vi "side_features - saveTxt.vi"() -> ()   [LabVIEW 2015]
uses:
  <vilib>/addons/_office/_exclsub.llb/font.ctl
  <vilib>/Analysis/baseanly.llb/Mean (DBL).vi
  <vilib>/Utility/file.llb/Read Delimited Spreadsheet (string).vi
  <vilib>/Utility/file.llb/Read From Spreadsheet File (string).vi
  <vilib>/addons/_office/NI_ReportGenerationToolkit.lvlib
  <vilib>/Utility/NIReport.llb/Excel/NI_Excel.lvclass
  <vilib>/vision/NI_Vision_Development_Module.lvlib
  TotalContoursConvexHull.dll
  <vilib>/Analysis/NI_AALBase.lvlib
  2-top_features_oilseed/HistProperty.dll
  PlantType.dll
panel:
  out "im_width":i32
  out "im_height":i32
  in  "The Path to save excel":path=path "E:/oilseed data/side_features"
  in  "Date Path":path=path "H:/oilseed data/date.txt"
  out "Current Path":path
  out "Current Number":string
  out "Rotated Image":T1(plugin-control)
  out "HistStat_whole":dbl[](array[numeric])
  out "PAR (perimeter-to-area ratio)":dbl
  out "SFD":sgl
  out "BW (minimum circumscribed box width)":dbl
  out "BH (minimum circumscribed box height)":dbl
  out "TPA (Total projective area)":dbl
  out "R (Rectangularity)":dbl
  out "IFD":sgl
  out "Hull area":dbl
  out "AC (Area Convexity)":dbl
  out "HWR":dbl
  in  "ROI_flower":T2={"Top"=0, "im_height"=1450, "L_left"=0, "im_width"=1680}
  out "NB (Number of blanchs)":i32
  out "FPAR (Flower perimeter-to-area ratio)":dbl
  out "FSFD":sgl
  out "FBW (Flower minimum circumscribed box width)":dbl
  out "FBH (Flower minimum circumscribed box height)":dbl
  out "YPA (Yellow projective area)":dbl
  out "FR (Flower rectangularity)":dbl
  out "FIFD":sgl
  out "FAC (Flower area Convexity)":dbl
  out "HistStat_flower":dbl[](array[numeric])
  in  "ROI_whole":T2={"Top"=90, "im_height"=1970, "L_left"=300, "im_width"=1450}
  out "FHWR":dbl
  out "GPA (Green projective area)":dbl
  out "GPAR (Green / Total)":dbl
  out "YPAR (Yellow / Total)":dbl
  out "Flower Hull Image":T1(plugin-control)
  out "Flower Hull Area":dbl
  out "Cropped Image":T1(plugin-control)
  out "Binary Image":T1(plugin-control)
  out "rgb Hull Image":T1(plugin-control)
  out "Flower Image (RGB)":T1(plugin-control)
  out "Flower Image (Label)":T1(plugin-control)
  out "PD1-6":sgl[](array[numeric])
  out "f array":dbl[](array[numeric])
  out "Combined Image":T1(plugin-control)
  in  "error in (no error) 2":errorcluster
  out "error out 2":errorcluster
  out "Image Path":path
  in  "Image Main Path":path=path "H:/oilseed data"
  out "error out":errorcluster
  in  "error in (no error)":errorcluster
  # "Digital evaluation software for oilseed rape phenotype-related traits (side-view) v1.0"
  # "测量数据"
  # "Whole plant"
  # "均值"
  # "标准差"
  # "平滑度"
  # "三阶矩"
  # "一致性"
  # "熵"
  # "Flower"
  # "Ratio"
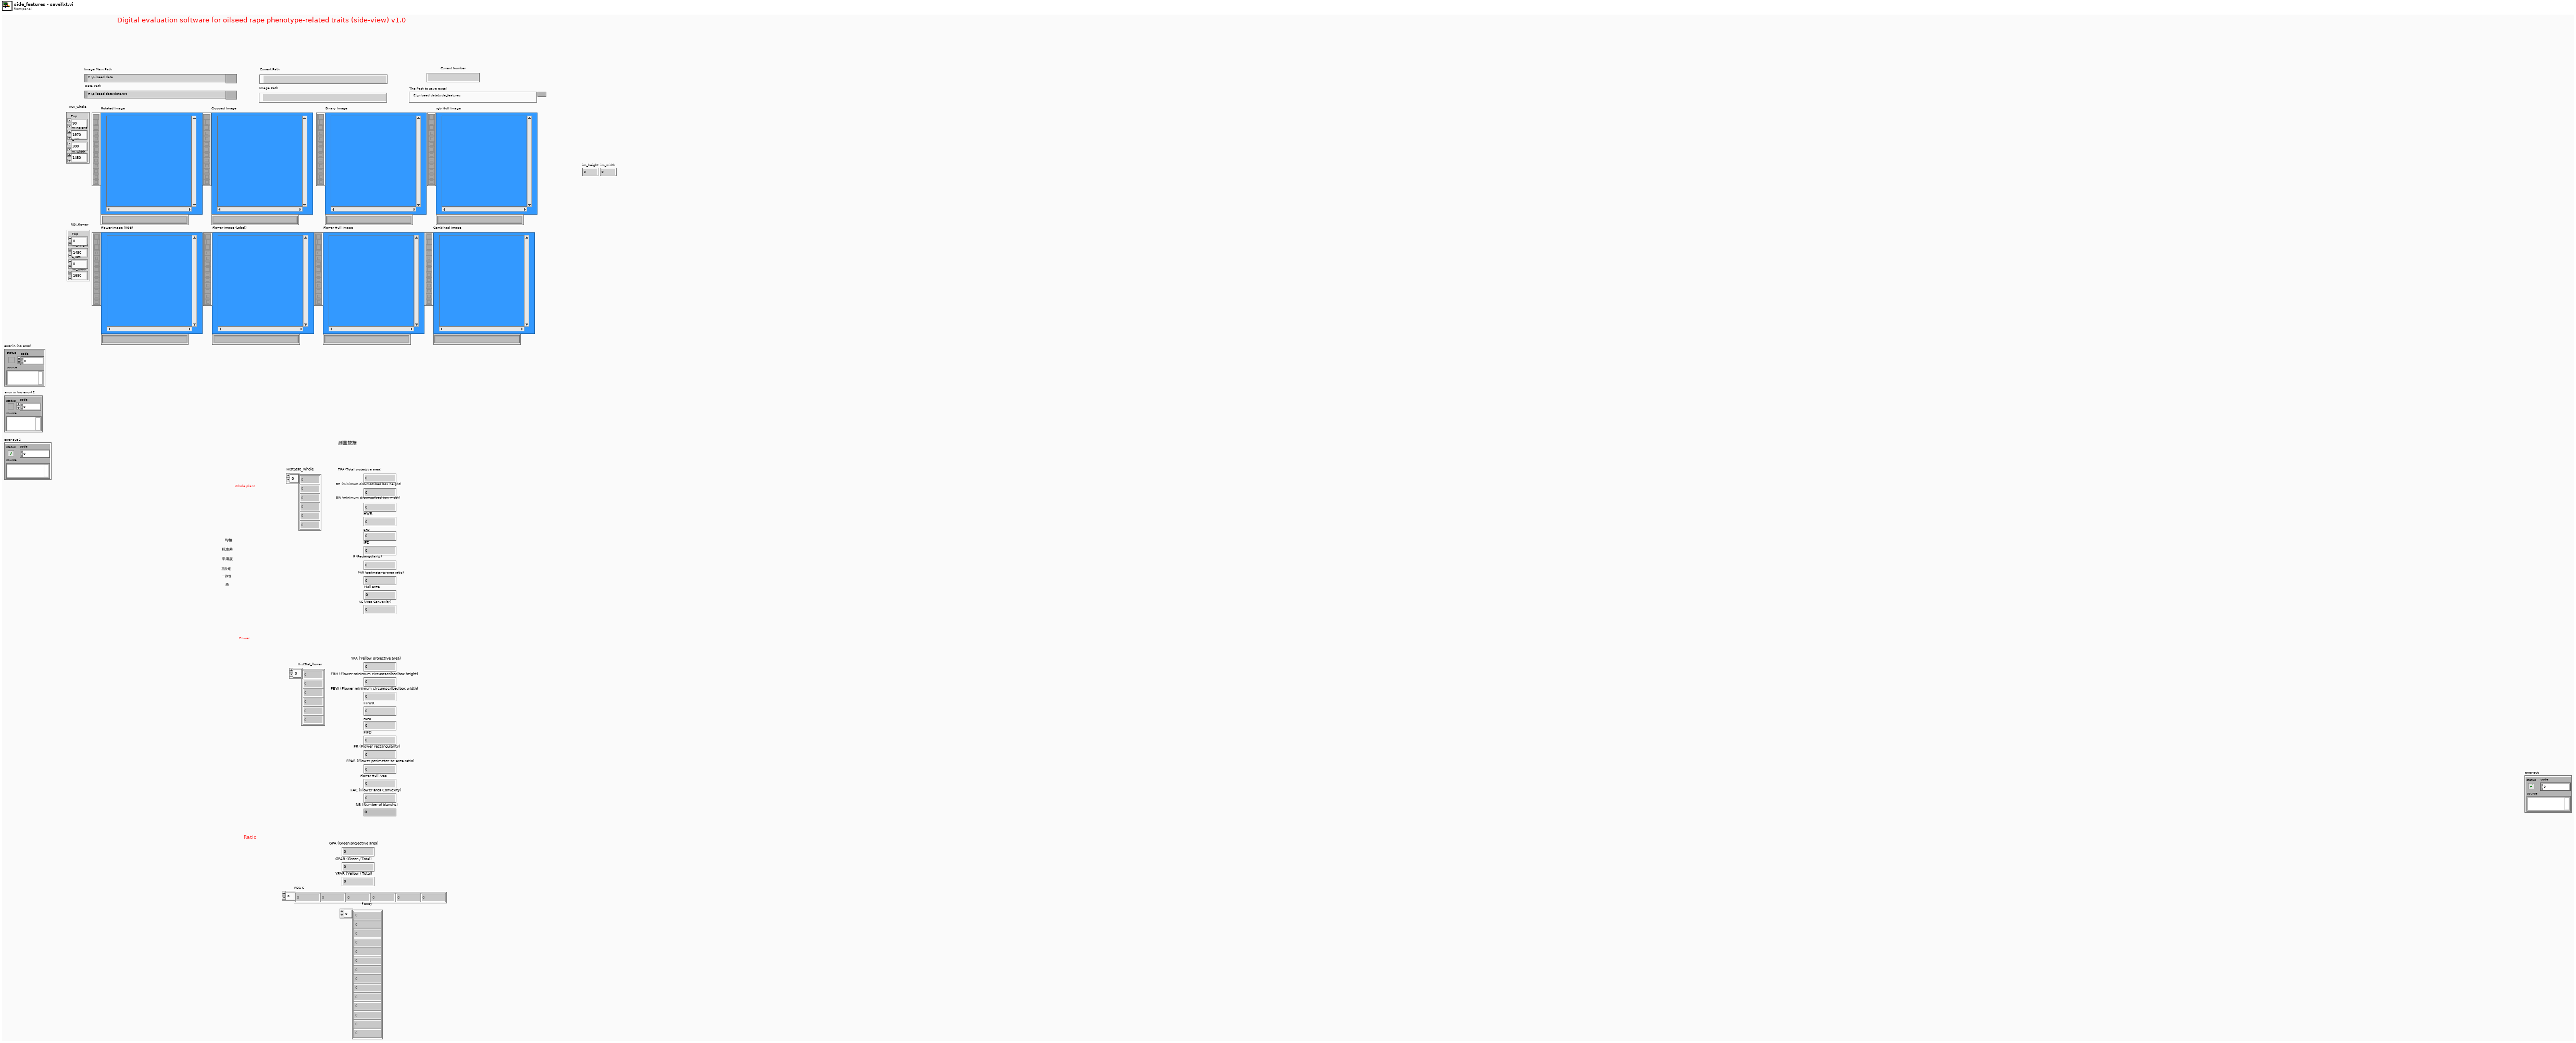
[diagram p1: front panel]
types:
  T1 = typedef "IMAQ Image.ctl" = refnum<image>
  T2 = cluster{"Top":i32, "im_height":i32, "L_left":i32, "im_width":i32}
  T3 = cluster{"report out":refnum<class "NI_report.lvclass">, "dup path":path}
  T4 = typedef "NI_ReportGenerationToolkit.lvlib/font.ctl" = cluster{"font name":string, "font size":dbl, "bold":u16, "italic":u16, "underline":u16, "strike through":u16, "font color":u32}
  T5 = typedef "Image Type" = u32
  T6 = typedef "Particle Parameters" = i32
  T7 = cluster{"String":string, "mean":dbl, "mean":dbl, "mean":dbl, "mean":dbl, "mean":dbl, "mean":dbl, "mean":dbl, "mean":dbl, "mean":dbl, "mean":dbl, "mean":dbl, "mean":dbl, "mean":dbl, "mean":dbl, "mean":dbl, "mean":dbl, "mean":dbl, "mean":dbl, "mean":dbl, "mean":dbl, "mean":dbl, "mean":dbl, "mean":dbl, "mean":dbl, "mean":dbl, "mean":dbl, "mean":dbl, "mean":dbl, "mean":dbl, "mean":dbl, "mean":dbl, "mean":dbl, "mean":dbl, "mean":dbl, "mean":dbl, "mean":dbl, "ratio":sgl[], "f array":dbl[]}
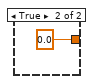
[diagram p2: hidden frame]
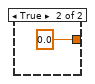
[diagram p3: hidden frame]
diagram:
  n1 = flat-sequence {
    tunnel: [w4] -> w1
    tunnel: w1 -> [w7]
    frame #0 {
      n2 = call "SheetInput (SubVI).vi"("error in (no error)"="error in (no error)", "The Path to save excel"="The Path to save excel") -> ("error out"=→"error out":errorcluster, "Cluster"=w4:T3)  [unwired: 8 in]
    }
    frame #1 {
      n3 = call-poly <vilib>:"Read Delimited Spreadsheet.vi"("file path (dialog if empty)"="Date Path") -> ("all rows"=w6:string[][])  [unwired: 9 in, 5 out]
      n4 = for {
        tunnel: "Image Main Path" -> [w19]
        tunnel: w6 -> [w17] mode=indexing
        tunnel: w7 -> [w11]
        n5 = Index Array(array=w17, index=0) -> (element=w12:string)
        n6 = Build Path(base path=w19, name or relative path=w12) -> (appended path=w13:path)
        "Image Path" <- w13
        n7 = Build Path(base path=w13, name or relative path="numbers.txt") -> (appended path=w15:path)
        n8 = call-poly <vilib>:"Read From Spreadsheet File.vi"("file path (dialog if empty)"=w15) -> ("all rows"=w14:string[][])  [unwired: 3 in, 7 out]
        n9 = for {
          tunnel: w13 -> [w542]
          tunnel: w14 -> [w543] mode=indexing
          tunnel: w11 -> [w450]
          shift-right: [w273] -> _
          shift-left: 2 -> [w84]
          w443 = 0
          w155 = T4 {"font name"="", "font size"=13.0, "bold"=0, "italic"=0, "underline"=0, "strike through"=0, "font color"=16777216} ("font")
          w534 = T5 0 items=["Grayscale (U8)", "Grayscale (I16)", "Grayscale (SGL)", "Complex (CSG)", "RGB (U32)", "HSL (U32)", "RGB (U64)", "Grayscale (U16)"] ("Image Type")
          n10 = Index Array(array=w543, index=0) -> (element=w541:string)
          n11 = local read "im_width"() -> (w24:i32)
          n12 = local read "im_height"() -> (w27:i32)
          n13 = local read "im_height"() -> (w26:i32)
          n14 = local read "im_width"() -> (w25:i32)
          n15 = call "IMAQ Create"("Image Name"="original", "Image Type"=w534) -> ("New Image"=w535:T1)  [unwired: 2 in, 2 out]
          n16 = call "IMAQ SetImageSize"("Y Resolution"=w26, "X Resolution"=w24, "Image"=w535) -> ("Image Out"=w533:T1)  [unwired: 1 in, 2 out]
          n17 = Initialize Array(sgl 0.0 ("element"), w27, w25) -> (w538:sgl[][])
          n18 = Increment(x=w84) -> (x+1=w273:i32)
          n19 = for {
            N: 15 -> [_]
            tunnel: w542 -> [w633]
            tunnel: w541 -> [w546]
            shift-right: [w599] -> w537
            shift-left: w538 -> [w602]
            shift-right: [w597] -> w458
            shift-left: w533 -> [w598]
            tunnel: [w595] -> w532 mode=indexing
            tunnel: [w594] -> w531 mode=indexing
            tunnel: [w593] -> w530 mode=indexing
            tunnel: [w592] -> w529 mode=indexing
            tunnel: [w591] -> w528 mode=indexing
            tunnel: [w590] -> w527 mode=indexing
            tunnel: [w589] -> w520 mode=indexing
            tunnel: [w588] -> w518 mode=indexing
            tunnel: [w587] -> w517 mode=indexing
            tunnel: [w586] -> w514 mode=indexing
            tunnel: [w585] -> w512 mode=indexing
            tunnel: [w584] -> w511 mode=indexing
            tunnel: [w583] -> w510 mode=indexing
            tunnel: [w582] -> w509 mode=indexing
            tunnel: [w581] -> w508 mode=indexing
            tunnel: [w580] -> w507 mode=indexing
            tunnel: [w578] -> w500 mode=indexing
            tunnel: [w577] -> w499 mode=indexing
            tunnel: [w576] -> w498 mode=indexing
            tunnel: [w575] -> w497 mode=indexing
            tunnel: [w574] -> w496 mode=indexing
            tunnel: [w573] -> w495 mode=indexing
            tunnel: [w554] -> w488 mode=indexing
            tunnel: [w572] -> w487 mode=indexing
            tunnel: [w571] -> w486 mode=indexing
            tunnel: [w570] -> w485 mode=indexing
            tunnel: [w569] -> w484 mode=indexing
            tunnel: [w568] -> w483 mode=indexing
            tunnel: [w567] -> w482 mode=indexing
            tunnel: [w566] -> w481 mode=indexing
            tunnel: [w553] -> w480 mode=indexing
            tunnel: [w552] -> w479 mode=indexing
            tunnel: [w565] -> w478 mode=indexing
            tunnel: [w564] -> w466 mode=indexing
            tunnel: [w563] -> w465 mode=indexing
            tunnel: [w562] -> w464 mode=indexing
            tunnel: [w546] -> w456 mode=indexing
            i -> [w545]
            w561 = T6[] [35] items=["Center of Mass X", "Center of Mass Y", "First Pixel X", "First Pixel Y", "Bounding Rect Left", "Bounding Rect Top", "Bounding Rect Right", "Bounding Rect Bottom", "Max Feret Diameter Start X", "Max Feret Diameter Start Y", "Max Feret Diameter End X", "Max Feret Diameter End Y", "Max Horiz. Segment Length Left", "Max Horiz. Segment Length Right", "Max Horiz. Segment Length Row", "-", "Bounding Rect Width", "Bounding Rect Height", "Bounding Rect Diagonal", "Perimeter", "Convex Hull Perimeter", "Holes' Perimeter", "Max Feret Diameter", "Equivalent Ellipse Major Axis", "Equivalent Ellipse Minor Axis", "Equivalent Ellipse Minor Axis (Feret)", "Equivalent Rect Long Side", "Equivalent Rect Short Side", "Equivalent Rect Diagonal", "Equivalent Rect Short Side (Feret)", "Average Horiz. Segment Length", "Average Vert. Segment Length", "Hydraulic Radius", "Waddel Disk Diameter", "-", "Area", "Holes' Area", "Particle & Holes' Area", "Convex Hull Area", "Image Area", "-", "Number of Holes", "Number of Horiz. Segments", "Number of Vert. Segments", "-", "Orientation", "Max Feret Diameter Orientation", "-", "% Area/Image Area", "% Area/(Particle & Holes' Area)", "Ratio of Equivalent Ellipse Axes", "Ratio of Equivalent Rect Sides", "-", "Elongation Factor", "Compactness Factor", "Heywood Circularity Factor", "Type Factor", "-", "Sum X", "Sum Y", "Sum XX", "Sum XY", "Sum YY", "Sum XXX", "Sum XXY", "Sum XYY", "Sum YYY", "-", "Moment of Inertia XX", "Moment of Inertia XY", "Moment of Inertia YY", "Moment of Inertia XXX", "Moment of Inertia XXY", "Moment of Inertia XYY", "Moment of Inertia YYY", "Norm. Moment of Inertia XX", "Norm. Moment of Inertia XY", "Norm. Moment of Inertia YY", "Norm. Moment of Inertia XXX", "Norm. Moment of Inertia XXY", "Norm. Moment of Inertia XYY", "Norm. Moment of Inertia YYY", "Hu Moment 1", "Hu Moment 2", "Hu Moment 3", "Hu Moment 4", "Hu Moment 5", "Hu Moment 6", "Hu Moment 7"] ("Pixel Measurements")
            w618 = u32 4 items=["Grayscale (U8)", "Grayscale (I16)", "Grayscale (SGL)", "Complex (CSG)", "RGB (U32)", "HSL (U32)", "RGB (U64)"] ("Image Type")
            w631 = T5 4 items=["Grayscale (U8)", "Grayscale (I16)", "Grayscale (SGL)", "Complex (CSG)", "RGB (U32)", "HSL (U32)", "RGB (U64)", "Grayscale (U16)"] ("Image Type")
            w638 = T5 4 items=["Grayscale (U8)", "Grayscale (I16)", "Grayscale (SGL)", "Complex (CSG)", "RGB (U32)", "HSL (U32)", "RGB (U64)", "Grayscale (U16)"] ("Image Type")
            n20 = Number To Decimal String(number=w545) -> (decimal integer string=w635:string)  [unwired: 1 out]
            n21 = Less Or Equal?(x=w545, y=u32 7) -> (x <= y?=w600:bool)
            n22 = Concatenate Strings(w546, "_" ("string"), w635, ".png" ("string")) -> (w627:string)
            "Current Number" <- w627
            n23 = call "IMAQ Create"("Image Name"="rgb", "Image Type"=w638) -> ("New Image"=w639:T1)  [unwired: 2 in, 2 out]
            n24 = Build Path(base path=w633, name or relative path=w627) -> (appended path=w634:path)
            "Current Path" <- w634
            n25 = call "IMAQ Create"("Image Name"="1", "Image Type"=w631) -> ("New Image"=w629:T1)  [unwired: 2 in, 2 out]
            n26 = call "IMAQ ReadFile"("File Path"=w634, "Image"=w639) -> ("Image Out"=w626:T1)  [unwired: 3 in, 6 out]
            n27 = call "IMAQ Rotate"("Maintain Size"=FALSE, "Angle (degrees)"=sgl 90.0, "Image Dst"=w629, "Image Src"=w626) -> ("Image Dst Out"=w616:T1)  [unwired: 4 in, 3 out]
            "Rotated Image" <- w616
            n28 = Unbundle By Name("ROI_whole") -> ("Top"=w622:i32, "im_height"=w623:i32, "L_left"=w624:i32, "im_width"=w625:i32)
            "im_height" <- w623
            "im_width" <- w625
            n29 = call "IMAQ ColorImageToArray"("Image"=w616) -> ("Image Pixels (U32)"=w621:u32[][])  [unwired: 2 in, 3 out]
            n30 = Array Subset(array=w621, index (row)=w622, length (row)=w623, index (col)=w624, length (col)=w625) -> (w620:u32[][])
            n31 = call "IMAQ Create"("Image Name"="ROI123", "Image Type"=w618) -> ("New Image"=w617:T1)  [unwired: 2 in, 2 out]
            n32 = call "IMAQ ArrayToColorImage"("Image Pixels (U32)"=w620, "Image"=w617) -> ("Image Out"=w551:T1)  [unwired: 2 in, 2 out]
            "Cropped Image" <- w551
            n33 = call "Flower segement(SubVI).vi"("Image in"=w551, "ROI 上半部分 2"="ROI_flower") -> ("黄色分量（油菜花）二值图"=w614:T1, "黄色分量（油菜花）"=→"Flower Image (RGB)":T1, "黄色分量（油菜花）Gray"=w604:T1, "Number of Particles"=w565:i32, "RGB花标记"=w547:T1)
            "NB (Number of blanchs)" <- w565
            "Flower Image (Label)" <- w547
            n34 = call "Segement(SubVI).vi"("Image in"=w551) -> ("Binary Image"=w550:T1)
            "Binary Image" <- w550
            n35 = call "IMAQ Particle Analysis"("Pixel Measurements"=w561, "Image"=w547) -> ("Particle Measurements (Pixels)"=w560:dbl[][])  [unwired: 3 in, 6 out]
            n36 = call "HistStat(SubVI).vi"("Binary Image"=w550, "Original Image"=w551) -> ("HistStat"=w596:dbl[])  [unwired: 1 out]
            "HistStat_whole" <- w596
            n37 = call "IMAQ ImageToArray"("Image"=w604) -> ("Image Pixels (U8)"=w605:u8[][])  [unwired: 2 in, 5 out]
            n38 = call "IMAQ GetImageSize"("Image"=w604) -> ("Y Resolution"=w608:i32, "X Resolution"=w609:i32)  [unwired: 1 in, 3 out]
            n39 = case shown="True" w600 {
              tunnel: w550 -> [_ w664]
              tunnel: w602 -> [w660 w663]
              tunnel: [w660 w662] -> w599
              frame False {
              }
              frame True {
                n40 = call "IMAQ ImageToArray"("Image"=w664) -> ("Image Pixels (U8)"=w667:u8[][])  [unwired: 2 in, 5 out]
                n41 = call "IMAQ GetImageSize"("Image"=w664) -> ("Y Resolution"=w665:i32, "X Resolution"=w666:i32)  [unwired: 1 in, 3 out]
                n42 = dll-call lib="H:/3-side_features_oilseed/PlantType.dll" fn="CalLeafDens"("bw"=w667, "row"=w665, "col"=w666, "GridSize"=5, "dens"=w663) -> ("dens"=w662:sgl[][])  [unwired: 7 in, 3 out]
              }
            }
            n43 = call "IMAQ Add"("Image Src A"=w598, "Image Src B"=w550) -> ("Image Dst Out"=w597:T1)  [unwired: 3 in, 3 out]
            n44 = Add Array Elements(numeric array=w560) -> (sum=w559:dbl)
            n45 = disable-structure shown="Enabled" {
              disable-tunnel: w605 -> [w672 w673]
              disable-tunnel: u8 8 ("y") -> [w671 _]
              disable-tunnel: [w668 w673] -> w607
              frame Enabled {
                n46 = Divide(x=w672, y=w671) -> (x/y=w670:dbl[][])
                n47 = Round Toward -Infinity(1:w670) -> (0:w669:dbl[][])
                n48 = To Unsigned Byte Integer(number=w669) -> (unsigned 8bit integer=w668:u8[][])
              }
              frame Disabled {
              }
            }
            n49 = Less Or Equal?(x=w559, y=50.0) -> (x <= y?=w557:bool)
            n50 = case shown="False" w557 {
              tunnel: w547 -> [w647 _]
              tunnel: [w646 0.0 ("areaSum")] -> w553
              frame False {
                w653 = T5 4 items=["Grayscale (U8)", "Grayscale (I16)", "Grayscale (SGL)", "Complex (CSG)", "RGB (U32)", "HSL (U32)", "RGB (U64)", "Grayscale (U16)"] ("Image Type")
                n51 = call "IMAQ ImageToArray"("Image"=w647) -> ("Image Pixels (U8)"=w658:u8[][])  [unwired: 2 in, 5 out]
                n52 = call "IMAQ GetImageSize"("Image"=w647) -> ("Y Resolution"=w656:i32, "X Resolution"=w657:i32)  [unwired: 1 in, 3 out]
                n53 = Initialize Array(u8 0 ("element"), w656, w657) -> (w648:u8[][])
                n54 = Initialize Array(u32 0 ("element"), w656, w657) -> (w651:u32[][])
                n55 = dll-call lib="H:/3-side_features_oilseed/TotalContoursConvexHull.dll" fn="TotalContoursConvexHull"("src"=w658, "width"=w657, "height"=w656, "bwhullimage"=w648, "rgbhullimage"=w651) -> ("areaSum"=w646:dbl, "rgbhullimage"=w654:u32[][])  [unwired: 7 in, 2 out]
                n56 = call "IMAQ Create"("Image Name"="rgbhullimage_flower", "Image Type"=w653) -> ("New Image"=w655:T1)  [unwired: 2 in, 2 out]
                n57 = call "IMAQ ArrayToColorImage"("Image Pixels (U32)"=w654, "Image"=w655) -> ("Image Out"=→"Flower Hull Image":T1)  [unwired: 2 in, 2 out]
              }
              frame True {
              }
            }
            "Flower Hull Area" <- w553
            n58 = Initialize Array(0.0 ("element"), 6 ("dimension size")) -> (w612:dbl[])
            n59 = dll-call lib="H:/2-top_features_oilseed/HistProperty.dll" fn="HistProperty"("Im"=w607, "row"=w608, "col"=w609, "G"=32, "HistStat"=w612) -> ("HistStat"=w579:dbl[])  [unwired: 7 in, 3 out]
            "HistStat_flower" <- w579
            n60 = call "Feature_flower(SubVI).vi"("黄色分量（油菜花）二值图"=w614) -> ("SF 3"=w567:dbl, "IFD 2"=w568:sgl, "SFD 2"=w569:sgl, "SH 2"=w572:dbl, "SW 2"=w571:dbl, "SE 2"=w566:dbl, "SA"=w554:dbl)  [unwired: 1 out]
            "FPAR (Flower perimeter-to-area ratio)" <- w566
            "FSFD" <- w569
            "FBW (Flower minimum circumscribed box width)" <- w571
            "FBH (Flower minimum circumscribed box height)" <- w572
            "YPA (Yellow projective area)" <- w554
            "FR (Flower rectangularity)" <- w567
            "FIFD" <- w568
            n61 = Equal?(x=w553, y=0.0) -> (x = y?=w556:bool)
            n62 = Divide(x=w572, y=w571) -> (x/y=w570:dbl)
            "FHWR" <- w570
            n63 = case shown="False" w556 {
              tunnel: w554 -> [w643 _]
              tunnel: w553 -> [w642 _]
              tunnel: [w641 0.0] -> w552
              frame False {
                n64 = Divide(x=w643, y=w642) -> (x/y=w641:dbl)
              }
              frame True {
              }
            }
            "FAC (Flower area Convexity)" <- w552
            n65 = call "Feature_whole(SubVI).vi"("Binary Image"=w550) -> ("SE"=w582:dbl, "rgb Hull Image 2"=→"rgb Hull Image":T1, "SA"=w589:dbl, "SFD"=w585:sgl, "Hull area"=w581:dbl, "SW"=w587:dbl, "SF 2"=w580:dbl, "IFD"=w584:sgl, "SF"=w583:dbl, "SH"=w588:dbl)  [unwired: 5 out]
            "PAR (perimeter-to-area ratio)" <- w582
            "SFD" <- w585
            "BW (minimum circumscribed box width)" <- w587
            "BH (minimum circumscribed box height)" <- w588
            "TPA (Total projective area)" <- w589
            "R (Rectangularity)" <- w583
            "IFD" <- w584
            "Hull area" <- w581
            "AC (Area Convexity)" <- w580
            n66 = Subtract(x=w589, y=w554) -> (x-y=w564:dbl)
            "GPA (Green projective area)" <- w564
            n67 = Divide(x=w554, y=w589) -> (x/y=w562:dbl)
            "YPAR (Yellow / Total)" <- w562
            n68 = Divide(x=w588, y=w587) -> (x/y=w586:dbl)
            "HWR" <- w586
            n69 = Divide(x=w564, y=w589) -> (x/y=w563:dbl)
            "GPAR (Green / Total)" <- w563
            n70 = Index Array(array=w596) -> (element #1=w595:dbl, element #2=w594:dbl, element #3=w593:dbl, element #4=w592:dbl, element #5=w591:dbl, element #6=w590:dbl)  [unwired: 6 in]
            n71 = Index Array(array=w579) -> (element #1=w578:dbl, element #2=w577:dbl, element #3=w576:dbl, element #4=w575:dbl, element #5=w574:dbl, element #6=w573:dbl)  [unwired: 6 in]
          }
          "Combined Image" <- w458
          n72 = call-poly <vilib>:"Mean.vi"("X"=w532) -> ("mean"=w526:dbl)  [unwired: 1 out]
          n73 = call-poly <vilib>:"Mean.vi"("X"=w531) -> ("mean"=w525:dbl)  [unwired: 1 out]
          n74 = call-poly <vilib>:"Mean.vi"("X"=w530) -> ("mean"=w524:dbl)  [unwired: 1 out]
          n75 = call-poly <vilib>:"Mean.vi"("X"=w529) -> ("mean"=w523:dbl)  [unwired: 1 out]
          n76 = call-poly <vilib>:"Mean.vi"("X"=w528) -> ("mean"=w522:dbl)  [unwired: 1 out]
          n77 = call-poly <vilib>:"Mean.vi"("X"=w527) -> ("mean"=w521:dbl)  [unwired: 1 out]
          n78 = call-poly <vilib>:"Mean.vi"("X"=w480) -> ("mean"=w469:dbl)  [unwired: 1 out]
          n79 = call-poly <vilib>:"Mean.vi"("X"=w479) -> ("mean"=w468:dbl)  [unwired: 1 out]
          n80 = call-poly <vilib>:"Mean.vi"("X"=w478) -> ("mean"=w467:dbl)  [unwired: 1 out]
          n81 = call-poly <vilib>:"Mean.vi"("X"=w500) -> ("mean"=w494:dbl)  [unwired: 1 out]
          n82 = call-poly <vilib>:"Mean.vi"("X"=w499) -> ("mean"=w493:dbl)  [unwired: 1 out]
          n83 = call-poly <vilib>:"Mean.vi"("X"=w498) -> ("mean"=w492:dbl)  [unwired: 1 out]
          n84 = call-poly <vilib>:"Mean.vi"("X"=w497) -> ("mean"=w491:dbl)  [unwired: 1 out]
          n85 = call-poly <vilib>:"Mean.vi"("X"=w496) -> ("mean"=w490:dbl)  [unwired: 1 out]
          n86 = call-poly <vilib>:"Mean.vi"("X"=w495) -> ("mean"=w489:dbl)  [unwired: 1 out]
          n87 = call-poly <vilib>:"Mean.vi"("X"=w486) -> ("mean"=w475:dbl)  [unwired: 1 out]
          n88 = call-poly <vilib>:"Mean.vi"("X"=w485) -> ("mean"=w474:dbl)  [unwired: 1 out]
          n89 = call-poly <vilib>:"Mean.vi"("X"=w487) -> ("mean"=w476:dbl)  [unwired: 1 out]
          n90 = call-poly <vilib>:"Mean.vi"("X"=w484) -> ("mean"=w473:dbl)  [unwired: 1 out]
          n91 = call-poly <vilib>:"Mean.vi"("X"=w482) -> ("mean"=w471:dbl)  [unwired: 1 out]
          n92 = call-poly <vilib>:"Mean.vi"("X"=w483) -> ("mean"=w472:dbl)  [unwired: 1 out]
          n93 = call-poly <vilib>:"Mean.vi"("X"=w481) -> ("mean"=w470:dbl)  [unwired: 1 out]
          n94 = call "RatioCalculation.vi"("dens"=w537) -> ("ratio"=w460:sgl[])  [unwired: 2 out]
          "PD1-6" <- w460
          n95 = call-poly <vilib>:"Mean.vi"("X"=w488) -> ("mean"=w477:dbl)  [unwired: 1 out]
          n96 = call-poly <vilib>:"Mean.vi"("X"=w466) -> ("mean"=w463:dbl)  [unwired: 1 out]
          n97 = call-poly <vilib>:"Mean.vi"("X"=w464) -> ("mean"=w461:dbl)  [unwired: 1 out]
          n98 = call-poly <vilib>:"Mean.vi"("X"=w509) -> ("mean"=w503:dbl)  [unwired: 1 out]
          n99 = call-poly <vilib>:"Mean.vi"("X"=w465) -> ("mean"=w462:dbl)  [unwired: 1 out]
          n100 = call-poly <vilib>:"Mean.vi"("X"=w520) -> ("mean"=w519:dbl)  [unwired: 1 out]
          n101 = call-poly <vilib>:"Mean.vi"("X"=w512) -> ("mean"=w506:dbl)  [unwired: 1 out]
          n102 = call-poly <vilib>:"Mean.vi"("X"=w517) -> ("mean"=w515:dbl)  [unwired: 1 out]
          n103 = call-poly <vilib>:"Mean.vi"("X"=w514) -> ("mean"=w513:dbl)  [unwired: 1 out]
          n104 = call-poly <vilib>:"Mean.vi"("X"=w518) -> ("mean"=w516:dbl)  [unwired: 1 out]
          n105 = call-poly <vilib>:"Mean.vi"("X"=w510) -> ("mean"=w504:dbl)  [unwired: 1 out]
          n106 = call-poly <vilib>:"Mean.vi"("X"=w511) -> ("mean"=w505:dbl)  [unwired: 1 out]
          n107 = call-poly <vilib>:"Mean.vi"("X"=w507) -> ("mean"=w501:dbl)  [unwired: 1 out]
          n108 = call-poly <vilib>:"Mean.vi"("X"=w508) -> ("mean"=w502:dbl)  [unwired: 1 out]
          n109 = call "FreqCalculation.vi"("Acc Image"=w458) -> ("f array"=w459:dbl[])  [unwired: 2 out]
          "f array" <- w459
          n110 = Index Array(array=w456, index=0) -> (element=w454:string)
          n111 = Bundle("String"=w454, "mean"=w526, "mean"=w525, "mean"=w524, "mean"=w523, "mean"=w522, "mean"=w521, "mean"=w519, "mean"=w516, "mean"=w515, "mean"=w513, "mean"=w506, "mean"=w505, "mean"=w504, "mean"=w503, "mean"=w502, "mean"=w501, "mean"=w494, "mean"=w493, "mean"=w492, "mean"=w491, "mean"=w490, "mean"=w489, "mean"=w477, "mean"=w476, "mean"=w475, "mean"=w474, "mean"=w473, "mean"=w472, "mean"=w471, "mean"=w470, "mean"=w469, "mean"=w468, "mean"=w467, "mean"=w463, "mean"=w462, "mean"=w461, "ratio"=w460, "f array"=w459) -> (w457:T7)  [unwired: 1 in]
          n112 = Bundle(w84, w443) -> (w452:cluster{i32, i32})  [unwired: 1 in]
          n113 = Unbundle(w450) -> ("report out"=w449:refnum<class "NI_report.lvclass">, "dup path"=w21:path)
          n114 = Unbundle(w457) -> ("String"=w453:string, "mean"=w447:dbl, "mean"=w428:dbl, "mean"=w426:dbl, "mean"=w424:dbl, "mean"=w422:dbl, "mean"=w420:dbl, "mean"=w418:dbl, "mean"=w351:dbl, "mean"=w350:dbl, "mean"=w349:dbl, "mean"=w348:dbl, "mean"=w345:dbl, "mean"=w344:dbl, "mean"=w343:dbl, "mean"=w342:dbl, "mean"=w341:dbl, "mean"=w340:dbl, "mean"=w339:dbl, "mean"=w338:dbl, "mean"=w337:dbl, "mean"=w332:dbl, "mean"=w331:dbl, "mean"=w330:dbl, "mean"=w264:dbl, "mean"=w263:dbl, "mean"=w262:dbl, "mean"=w261:dbl, "mean"=w260:dbl, "mean"=w259:dbl, "mean"=w258:dbl, "mean"=w257:dbl, "mean"=w256:dbl, "mean"=w255:dbl, "mean"=w254:dbl, "mean"=w253:dbl, "mean"=w252:dbl, "ratio"=w232:sgl[], "f array"=w216:dbl[])
          n115 = Increment(x=w443) -> (x+1=w410:i32)
          n116 = Index Array(array=w232, index=5) -> (element=w231:sgl)
          n117 = Index Array(array=w232, index=4) -> (element=w233:sgl)
          n118 = Index Array(array=w232, index=3) -> (element=w236:sgl)
          n119 = Index Array(array=w232, index=2) -> (element=w243:sgl)
          n120 = Index Array(array=w232, index=1) -> (element=w244:sgl)
          n121 = Index Array(array=w232, index=0) -> (element=w250:sgl)
          n122 = Index Array(array=w216, index=9) -> (element=w145:dbl)
          n123 = Index Array(array=w216, index=8) -> (element=w146:dbl)
          n124 = Index Array(array=w216, index=7) -> (element=w147:dbl)
          n125 = Index Array(array=w216, index=6) -> (element=w148:dbl)
          n126 = Index Array(array=w216, index=5) -> (element=w149:dbl)
          n127 = Index Array(array=w216, index=4) -> (element=w150:dbl)
          n128 = Index Array(array=w216, index=3) -> (element=w151:dbl)
          n129 = Index Array(array=w216, index=2) -> (element=w152:dbl)
          n130 = Index Array(array=w216, index=1) -> (element=w153:dbl)
          n131 = Index Array(array=w216, index=0) -> (element=w154:dbl)
          n132 = Index Array(array=w216, index=13) -> (element=w141:dbl)
          n133 = Index Array(array=w216, index=12) -> (element=w142:dbl)
          n134 = Index Array(array=w216, index=11) -> (element=w143:dbl)
          n135 = Index Array(array=w216, index=10) -> (element=w144:dbl)
          n136 = call <vilib>:"Excel Easy Text.vi"("report in"=w449, "border? (F)"=FALSE, "font"=w155, "text"=w453, "start (-1, -1)"=w452, "error in (no error)"="error in (no error) 2") -> ("report out"=w444:refnum<class "NI_report.lvclass">, "error out"=w441:errorcluster)  [unwired: 5 in, 3 out]
          n137 = Bundle(w84, w410) -> (w442:cluster{i32, i32})  [unwired: 1 in]
          n138 = Number To Fractional String(number=w447) -> (F-format string=w446:string)  [unwired: 3 in]
          n139 = Increment(x=w410) -> (x+1=w138:i32)
          n140 = call <vilib>:"Excel Easy Text.vi"("report in"=w444, "border? (F)"=FALSE, "font"=w155, "text"=w446, "start (-1, -1)"=w442, "error in (no error)"=w441) -> ("report out"=w434:refnum<class "NI_report.lvclass">, "error out"=w440:errorcluster)  [unwired: 5 in, 3 out]
          n141 = Bundle(w84, w138) -> (w409:cluster{i32, i32})  [unwired: 1 in]
          n142 = Number To Fractional String(number=w428) -> (F-format string=w427:string)  [unwired: 3 in]
          n143 = Increment(x=w138) -> (x+1=w137:i32)
          n144 = call <vilib>:"Excel Easy Text.vi"("report in"=w434, "border? (F)"=FALSE, "font"=w155, "text"=w427, "start (-1, -1)"=w409, "error in (no error)"=w440) -> ("report out"=w433:refnum<class "NI_report.lvclass">, "error out"=w439:errorcluster)  [unwired: 5 in, 3 out]
          n145 = Bundle(w84, w137) -> (w81:cluster{i32, i32})  [unwired: 1 in]
          n146 = Number To Fractional String(number=w426) -> (F-format string=w425:string)  [unwired: 3 in]
          n147 = Increment(x=w137) -> (x+1=w136:i32)
          n148 = call <vilib>:"Excel Easy Text.vi"("report in"=w433, "border? (F)"=FALSE, "font"=w155, "text"=w425, "start (-1, -1)"=w81, "error in (no error)"=w439) -> ("report out"=w432:refnum<class "NI_report.lvclass">, "error out"=w438:errorcluster)  [unwired: 5 in, 3 out]
          n149 = Bundle(w84, w136) -> (w80:cluster{i32, i32})  [unwired: 1 in]
          n150 = Number To Fractional String(number=w424) -> (F-format string=w423:string)  [unwired: 3 in]
          n151 = Increment(x=w136) -> (x+1=w135:i32)
          n152 = call <vilib>:"Excel Easy Text.vi"("report in"=w432, "border? (F)"=FALSE, "font"=w155, "text"=w423, "start (-1, -1)"=w80, "error in (no error)"=w438) -> ("report out"=w431:refnum<class "NI_report.lvclass">, "error out"=w437:errorcluster)  [unwired: 5 in, 3 out]
          n153 = Bundle(w84, w135) -> (w79:cluster{i32, i32})  [unwired: 1 in]
          n154 = Number To Fractional String(number=w422) -> (F-format string=w421:string)  [unwired: 3 in]
          n155 = Increment(x=w135) -> (x+1=w134:i32)
          n156 = call <vilib>:"Excel Easy Text.vi"("report in"=w431, "border? (F)"=FALSE, "font"=w155, "text"=w421, "start (-1, -1)"=w79, "error in (no error)"=w437) -> ("report out"=w430:refnum<class "NI_report.lvclass">, "error out"=w436:errorcluster)  [unwired: 5 in, 3 out]
          n157 = Bundle(w84, w134) -> (w78:cluster{i32, i32})  [unwired: 1 in]
          n158 = Number To Fractional String(number=w420) -> (F-format string=w419:string)  [unwired: 3 in]
          n159 = Increment(x=w134) -> (x+1=w133:i32)
          n160 = call <vilib>:"Excel Easy Text.vi"("report in"=w430, "border? (F)"=FALSE, "font"=w155, "text"=w419, "start (-1, -1)"=w78, "error in (no error)"=w436) -> ("report out"=w429:refnum<class "NI_report.lvclass">, "error out"=w435:errorcluster)  [unwired: 5 in, 3 out]
          n161 = Bundle(w84, w133) -> (w77:cluster{i32, i32})  [unwired: 1 in]
          n162 = Number To Fractional String(number=w418) -> (F-format string=w417:string)  [unwired: 3 in]
          n163 = Increment(x=w133) -> (x+1=w132:i32)
          n164 = call <vilib>:"Excel Easy Text.vi"("report in"=w429, "border? (F)"=FALSE, "font"=w155, "text"=w417, "start (-1, -1)"=w77, "error in (no error)"=w435) -> ("report out"=w353:refnum<class "NI_report.lvclass">, "error out"=w352:errorcluster)  [unwired: 5 in, 3 out]
          n165 = Bundle(w84, w132) -> (w76:cluster{i32, i32})  [unwired: 1 in]
          n166 = Number To Fractional String(number=w351) -> (F-format string=w402:string)  [unwired: 3 in]
          n167 = Increment(x=w132) -> (x+1=w131:i32)
          n168 = call <vilib>:"Excel Easy Text.vi"("report in"=w353, "border? (F)"=FALSE, "font"=w155, "text"=w402, "start (-1, -1)"=w76, "error in (no error)"=w352) -> ("report out"=w405:refnum<class "NI_report.lvclass">, "error out"=w408:errorcluster)  [unwired: 5 in, 3 out]
          n169 = Bundle(w84, w131) -> (w75:cluster{i32, i32})  [unwired: 1 in]
          n170 = Number To Fractional String(number=w350) -> (F-format string=w401:string)  [unwired: 3 in]
          n171 = Increment(x=w131) -> (x+1=w130:i32)
          n172 = call <vilib>:"Excel Easy Text.vi"("report in"=w405, "border? (F)"=FALSE, "font"=w155, "text"=w401, "start (-1, -1)"=w75, "error in (no error)"=w408) -> ("report out"=w404:refnum<class "NI_report.lvclass">, "error out"=w407:errorcluster)  [unwired: 5 in, 3 out]
          n173 = Bundle(w84, w130) -> (w74:cluster{i32, i32})  [unwired: 1 in]
          n174 = Number To Fractional String(number=w349) -> (F-format string=w400:string)  [unwired: 3 in]
          n175 = Increment(x=w130) -> (x+1=w129:i32)
          n176 = call <vilib>:"Excel Easy Text.vi"("report in"=w404, "border? (F)"=FALSE, "font"=w155, "text"=w400, "start (-1, -1)"=w74, "error in (no error)"=w407) -> ("report out"=w403:refnum<class "NI_report.lvclass">, "error out"=w406:errorcluster)  [unwired: 5 in, 3 out]
          n177 = Bundle(w84, w129) -> (w73:cluster{i32, i32})  [unwired: 1 in]
          n178 = Number To Fractional String(number=w348) -> (F-format string=w399:string)  [unwired: 3 in]
          n179 = Increment(x=w129) -> (x+1=w128:i32)
          n180 = call <vilib>:"Excel Easy Text.vi"("report in"=w403, "border? (F)"=FALSE, "font"=w155, "text"=w399, "start (-1, -1)"=w73, "error in (no error)"=w406) -> ("report out"=w347:refnum<class "NI_report.lvclass">, "error out"=w346:errorcluster)  [unwired: 5 in, 3 out]
          n181 = Bundle(w84, w128) -> (w72:cluster{i32, i32})  [unwired: 1 in]
          n182 = Number To Fractional String(number=w345) -> (F-format string=w388:string)  [unwired: 3 in]
          n183 = Increment(x=w128) -> (x+1=w127:i32)
          n184 = call <vilib>:"Excel Easy Text.vi"("report in"=w347, "border? (F)"=FALSE, "font"=w155, "text"=w388, "start (-1, -1)"=w72, "error in (no error)"=w346) -> ("report out"=w391:refnum<class "NI_report.lvclass">, "error out"=w394:errorcluster)  [unwired: 5 in, 3 out]
          n185 = Bundle(w84, w127) -> (w71:cluster{i32, i32})  [unwired: 1 in]
          n186 = Number To Fractional String(number=w344) -> (F-format string=w387:string)  [unwired: 3 in]
          n187 = Increment(x=w127) -> (x+1=w126:i32)
          n188 = call <vilib>:"Excel Easy Text.vi"("report in"=w391, "border? (F)"=FALSE, "font"=w155, "text"=w387, "start (-1, -1)"=w71, "error in (no error)"=w394) -> ("report out"=w390:refnum<class "NI_report.lvclass">, "error out"=w393:errorcluster)  [unwired: 5 in, 3 out]
          n189 = Bundle(w84, w126) -> (w70:cluster{i32, i32})  [unwired: 1 in]
          n190 = Number To Fractional String(number=w343) -> (F-format string=w386:string)  [unwired: 3 in]
          n191 = Increment(x=w126) -> (x+1=w125:i32)
          n192 = call <vilib>:"Excel Easy Text.vi"("report in"=w390, "border? (F)"=FALSE, "font"=w155, "text"=w386, "start (-1, -1)"=w70, "error in (no error)"=w393) -> ("report out"=w389:refnum<class "NI_report.lvclass">, "error out"=w392:errorcluster)  [unwired: 5 in, 3 out]
          n193 = Bundle(w84, w125) -> (w69:cluster{i32, i32})  [unwired: 1 in]
          n194 = Number To Fractional String(number=w342) -> (F-format string=w385:string)  [unwired: 3 in]
          n195 = Increment(x=w125) -> (x+1=w123:i32)
          n196 = call <vilib>:"Excel Easy Text.vi"("report in"=w389, "border? (F)"=FALSE, "font"=w155, "text"=w385, "start (-1, -1)"=w69, "error in (no error)"=w392) -> ("report out"=w336:refnum<class "NI_report.lvclass">, "error out"=w335:errorcluster)  [unwired: 5 in, 3 out]
          n197 = Bundle(w84, w123) -> (w68:cluster{i32, i32})  [unwired: 1 in]
          n198 = Number To Fractional String(number=w341) -> (F-format string=w374:string)  [unwired: 3 in]
          n199 = Increment(x=w123) -> (x+1=w122:i32)
          n200 = call <vilib>:"Excel Easy Text.vi"("report in"=w336, "border? (F)"=FALSE, "font"=w155, "text"=w374, "start (-1, -1)"=w68, "error in (no error)"=w335) -> ("report out"=w377:refnum<class "NI_report.lvclass">, "error out"=w380:errorcluster)  [unwired: 5 in, 3 out]
          n201 = Bundle(w84, w122) -> (w67:cluster{i32, i32})  [unwired: 1 in]
          n202 = Number To Fractional String(number=w340) -> (F-format string=w373:string)  [unwired: 3 in]
          n203 = Increment(x=w122) -> (x+1=w121:i32)
          n204 = call <vilib>:"Excel Easy Text.vi"("report in"=w377, "border? (F)"=FALSE, "font"=w155, "text"=w373, "start (-1, -1)"=w67, "error in (no error)"=w380) -> ("report out"=w376:refnum<class "NI_report.lvclass">, "error out"=w379:errorcluster)  [unwired: 5 in, 3 out]
          n205 = Bundle(w84, w121) -> (w66:cluster{i32, i32})  [unwired: 1 in]
          n206 = Number To Fractional String(number=w339) -> (F-format string=w372:string)  [unwired: 3 in]
          n207 = Increment(x=w121) -> (x+1=w120:i32)
          n208 = call <vilib>:"Excel Easy Text.vi"("report in"=w376, "border? (F)"=FALSE, "font"=w155, "text"=w372, "start (-1, -1)"=w66, "error in (no error)"=w379) -> ("report out"=w375:refnum<class "NI_report.lvclass">, "error out"=w378:errorcluster)  [unwired: 5 in, 3 out]
          n209 = Bundle(w84, w120) -> (w65:cluster{i32, i32})  [unwired: 1 in]
          n210 = Number To Fractional String(number=w338) -> (F-format string=w371:string)  [unwired: 3 in]
          n211 = Increment(x=w120) -> (x+1=w119:i32)
          n212 = call <vilib>:"Excel Easy Text.vi"("report in"=w375, "border? (F)"=FALSE, "font"=w155, "text"=w371, "start (-1, -1)"=w65, "error in (no error)"=w378) -> ("report out"=w334:refnum<class "NI_report.lvclass">, "error out"=w333:errorcluster)  [unwired: 5 in, 3 out]
          n213 = Bundle(w84, w119) -> (w64:cluster{i32, i32})  [unwired: 1 in]
          n214 = Number To Fractional String(number=w337) -> (F-format string=w361:string)  [unwired: 3 in]
          n215 = Increment(x=w119) -> (x+1=w118:i32)
          n216 = call <vilib>:"Excel Easy Text.vi"("report in"=w334, "border? (F)"=FALSE, "font"=w155, "text"=w361, "start (-1, -1)"=w64, "error in (no error)"=w333) -> ("report out"=w364:refnum<class "NI_report.lvclass">, "error out"=w367:errorcluster)  [unwired: 5 in, 3 out]
          n217 = Bundle(w84, w118) -> (w63:cluster{i32, i32})  [unwired: 1 in]
          n218 = Number To Fractional String(number=w332) -> (F-format string=w360:string)  [unwired: 3 in]
          n219 = Increment(x=w118) -> (x+1=w117:i32)
          n220 = call <vilib>:"Excel Easy Text.vi"("report in"=w364, "border? (F)"=FALSE, "font"=w155, "text"=w360, "start (-1, -1)"=w63, "error in (no error)"=w367) -> ("report out"=w363:refnum<class "NI_report.lvclass">, "error out"=w366:errorcluster)  [unwired: 5 in, 3 out]
          n221 = Bundle(w84, w117) -> (w62:cluster{i32, i32})  [unwired: 1 in]
          n222 = Number To Fractional String(number=w331) -> (F-format string=w359:string)  [unwired: 3 in]
          n223 = Increment(x=w117) -> (x+1=w116:i32)
          n224 = call <vilib>:"Excel Easy Text.vi"("report in"=w363, "border? (F)"=FALSE, "font"=w155, "text"=w359, "start (-1, -1)"=w62, "error in (no error)"=w366) -> ("report out"=w362:refnum<class "NI_report.lvclass">, "error out"=w365:errorcluster)  [unwired: 5 in, 3 out]
          n225 = Bundle(w84, w116) -> (w61:cluster{i32, i32})  [unwired: 1 in]
          n226 = Number To Fractional String(number=w330) -> (F-format string=w358:string)  [unwired: 3 in]
          n227 = Increment(x=w116) -> (x+1=w115:i32)
          n228 = call <vilib>:"Excel Easy Text.vi"("report in"=w362, "border? (F)"=FALSE, "font"=w155, "text"=w358, "start (-1, -1)"=w61, "error in (no error)"=w365) -> ("report out"=w272:refnum<class "NI_report.lvclass">, "error out"=w271:errorcluster)  [unwired: 5 in, 3 out]
          n229 = Bundle(w84, w115) -> (w60:cluster{i32, i32})  [unwired: 1 in]
          n230 = Number To Fractional String(number=w264) -> (F-format string=w323:string)  [unwired: 3 in]
          n231 = Increment(x=w115) -> (x+1=w114:i32)
          n232 = call <vilib>:"Excel Easy Text.vi"("report in"=w272, "border? (F)"=FALSE, "font"=w155, "text"=w323, "start (-1, -1)"=w60, "error in (no error)"=w271) -> ("report out"=w326:refnum<class "NI_report.lvclass">, "error out"=w329:errorcluster)  [unwired: 5 in, 3 out]
          n233 = Bundle(w84, w114) -> (w59:cluster{i32, i32})  [unwired: 1 in]
          n234 = Number To Fractional String(number=w263) -> (F-format string=w322:string)  [unwired: 3 in]
          n235 = Increment(x=w114) -> (x+1=w113:i32)
          n236 = call <vilib>:"Excel Easy Text.vi"("report in"=w326, "border? (F)"=FALSE, "font"=w155, "text"=w322, "start (-1, -1)"=w59, "error in (no error)"=w329) -> ("report out"=w325:refnum<class "NI_report.lvclass">, "error out"=w328:errorcluster)  [unwired: 5 in, 3 out]
          n237 = Bundle(w84, w113) -> (w58:cluster{i32, i32})  [unwired: 1 in]
          n238 = Number To Fractional String(number=w262) -> (F-format string=w321:string)  [unwired: 3 in]
          n239 = Increment(x=w113) -> (x+1=w112:i32)
          n240 = call <vilib>:"Excel Easy Text.vi"("report in"=w325, "border? (F)"=FALSE, "font"=w155, "text"=w321, "start (-1, -1)"=w58, "error in (no error)"=w328) -> ("report out"=w324:refnum<class "NI_report.lvclass">, "error out"=w327:errorcluster)  [unwired: 5 in, 3 out]
          n241 = Bundle(w84, w112) -> (w57:cluster{i32, i32})  [unwired: 1 in]
          n242 = Number To Fractional String(number=w261) -> (F-format string=w320:string)  [unwired: 3 in]
          n243 = Increment(x=w112) -> (x+1=w111:i32)
          n244 = call <vilib>:"Excel Easy Text.vi"("report in"=w324, "border? (F)"=FALSE, "font"=w155, "text"=w320, "start (-1, -1)"=w57, "error in (no error)"=w327) -> ("report out"=w270:refnum<class "NI_report.lvclass">, "error out"=w269:errorcluster)  [unwired: 5 in, 3 out]
          n245 = Bundle(w84, w111) -> (w56:cluster{i32, i32})  [unwired: 1 in]
          n246 = Number To Fractional String(number=w260) -> (F-format string=w309:string)  [unwired: 3 in]
          n247 = Increment(x=w111) -> (x+1=w110:i32)
          n248 = call <vilib>:"Excel Easy Text.vi"("report in"=w270, "border? (F)"=FALSE, "font"=w155, "text"=w309, "start (-1, -1)"=w56, "error in (no error)"=w269) -> ("report out"=w312:refnum<class "NI_report.lvclass">, "error out"=w315:errorcluster)  [unwired: 5 in, 3 out]
          n249 = Bundle(w84, w110) -> (w55:cluster{i32, i32})  [unwired: 1 in]
          n250 = Number To Fractional String(number=w259) -> (F-format string=w308:string)  [unwired: 3 in]
          n251 = Increment(x=w110) -> (x+1=w109:i32)
          n252 = call <vilib>:"Excel Easy Text.vi"("report in"=w312, "border? (F)"=FALSE, "font"=w155, "text"=w308, "start (-1, -1)"=w55, "error in (no error)"=w315) -> ("report out"=w311:refnum<class "NI_report.lvclass">, "error out"=w314:errorcluster)  [unwired: 5 in, 3 out]
          n253 = Bundle(w84, w109) -> (w54:cluster{i32, i32})  [unwired: 1 in]
          n254 = Number To Fractional String(number=w258) -> (F-format string=w307:string)  [unwired: 3 in]
          n255 = Increment(x=w109) -> (x+1=w108:i32)
          n256 = call <vilib>:"Excel Easy Text.vi"("report in"=w311, "border? (F)"=FALSE, "font"=w155, "text"=w307, "start (-1, -1)"=w54, "error in (no error)"=w314) -> ("report out"=w310:refnum<class "NI_report.lvclass">, "error out"=w313:errorcluster)  [unwired: 5 in, 3 out]
          n257 = Bundle(w84, w108) -> (w53:cluster{i32, i32})  [unwired: 1 in]
          n258 = Number To Fractional String(number=w257) -> (F-format string=w306:string)  [unwired: 3 in]
          n259 = Increment(x=w108) -> (x+1=w107:i32)
          n260 = call <vilib>:"Excel Easy Text.vi"("report in"=w310, "border? (F)"=FALSE, "font"=w155, "text"=w306, "start (-1, -1)"=w53, "error in (no error)"=w313) -> ("report out"=w268:refnum<class "NI_report.lvclass">, "error out"=w267:errorcluster)  [unwired: 5 in, 3 out]
          n261 = Bundle(w84, w107) -> (w52:cluster{i32, i32})  [unwired: 1 in]
          n262 = Increment(x=w107) -> (x+1=w106:i32)
          n263 = Number To Fractional String(number=w256) -> (F-format string=w295:string)  [unwired: 3 in]
          n264 = Bundle(w84, w106) -> (w51:cluster{i32, i32})  [unwired: 1 in]
          n265 = Number To Fractional String(number=w255) -> (F-format string=w294:string)  [unwired: 3 in]
          n266 = call <vilib>:"Excel Easy Text.vi"("report in"=w268, "border? (F)"=FALSE, "text"=w295, "start (-1, -1)"=w52, "error in (no error)"=w267) -> ("report out"=w298:refnum<class "NI_report.lvclass">, "error out"=w301:errorcluster)  [unwired: 6 in, 3 out]
          n267 = Increment(x=w106) -> (x+1=w105:i32)
          n268 = call <vilib>:"Excel Easy Text.vi"("report in"=w298, "border? (F)"=FALSE, "font"=w155, "text"=w294, "start (-1, -1)"=w51, "error in (no error)"=w301) -> ("report out"=w297:refnum<class "NI_report.lvclass">, "error out"=w300:errorcluster)  [unwired: 5 in, 3 out]
          n269 = Bundle(w84, w105) -> (w50:cluster{i32, i32})  [unwired: 1 in]
          n270 = Number To Fractional String(number=w254) -> (F-format string=w293:string)  [unwired: 3 in]
          n271 = Increment(x=w105) -> (x+1=w104:i32)
          n272 = call <vilib>:"Excel Easy Text.vi"("report in"=w297, "border? (F)"=FALSE, "font"=w155, "text"=w293, "start (-1, -1)"=w50, "error in (no error)"=w300) -> ("report out"=w296:refnum<class "NI_report.lvclass">, "error out"=w299:errorcluster)  [unwired: 5 in, 3 out]
          n273 = Bundle(w84, w104) -> (w49:cluster{i32, i32})  [unwired: 1 in]
          n274 = Number To Fractional String(number=w253) -> (F-format string=w292:string)  [unwired: 3 in]
          n275 = Increment(x=w104) -> (x+1=w103:i32)
          n276 = call <vilib>:"Excel Easy Text.vi"("report in"=w296, "border? (F)"=FALSE, "font"=w155, "text"=w292, "start (-1, -1)"=w49, "error in (no error)"=w299) -> ("report out"=w266:refnum<class "NI_report.lvclass">, "error out"=w265:errorcluster)  [unwired: 5 in, 3 out]
          n277 = Bundle(w84, w103) -> (w48:cluster{i32, i32})  [unwired: 1 in]
          n278 = Number To Fractional String(number=w252) -> (F-format string=w281:string)  [unwired: 3 in]
          n279 = Increment(x=w103) -> (x+1=w102:i32)
          n280 = call <vilib>:"Excel Easy Text.vi"("report in"=w266, "border? (F)"=FALSE, "font"=w155, "text"=w281, "start (-1, -1)"=w48, "error in (no error)"=w265) -> ("report out"=w284:refnum<class "NI_report.lvclass">, "error out"=w287:errorcluster)  [unwired: 5 in, 3 out]
          n281 = Bundle(w84, w102) -> (w47:cluster{i32, i32})  [unwired: 1 in]
          n282 = Increment(x=w102) -> (x+1=w101:i32)
          n283 = Number To Fractional String(number=w250) -> (F-format string=w280:string)  [unwired: 3 in]
          n284 = Increment(x=w101) -> (x+1=w100:i32)
          n285 = call <vilib>:"Excel Easy Text.vi"("report in"=w284, "border? (F)"=FALSE, "font"=w155, "text"=w280, "start (-1, -1)"=w47, "error in (no error)"=w287) -> ("report out"=w283:refnum<class "NI_report.lvclass">, "error out"=w286:errorcluster)  [unwired: 5 in, 3 out]
          n286 = Bundle(w84, w100) -> (w28:cluster{i32, i32})  [unwired: 1 in]
          n287 = Bundle(w84, w101) -> (w46:cluster{i32, i32})  [unwired: 1 in]
          n288 = Number To Fractional String(number=w244) -> (F-format string=w279:string)  [unwired: 3 in]
          n289 = call <vilib>:"Excel Easy Text.vi"("report in"=w283, "border? (F)"=FALSE, "font"=w155, "text"=w279, "start (-1, -1)"=w46, "error in (no error)"=w286) -> ("report out"=w282:refnum<class "NI_report.lvclass">, "error out"=w285:errorcluster)  [unwired: 5 in, 3 out]
          n290 = Number To Fractional String(number=w243) -> (F-format string=w278:string)  [unwired: 3 in]
          n291 = Increment(x=w100) -> (x+1=w99:i32)
          n292 = call <vilib>:"Excel Easy Text.vi"("report in"=w282, "border? (F)"=FALSE, "font"=w155, "text"=w278, "start (-1, -1)"=w28, "error in (no error)"=w285) -> ("report out"=w235:refnum<class "NI_report.lvclass">, "error out"=w234:errorcluster)  [unwired: 5 in, 3 out]
          n293 = Bundle(w84, w99) -> (w45:cluster{i32, i32})  [unwired: 1 in]
          n294 = Number To Fractional String(number=w236) -> (F-format string=w242:string)  [unwired: 3 in]
          n295 = Increment(x=w99) -> (x+1=w98:i32)
          n296 = call <vilib>:"Excel Easy Text.vi"("report in"=w235, "border? (F)"=FALSE, "font"=w155, "text"=w242, "start (-1, -1)"=w45, "error in (no error)"=w234) -> ("report out"=w200:refnum<class "NI_report.lvclass">, "error out"=w199:errorcluster)  [unwired: 5 in, 3 out]
          n297 = Bundle(w84, w98) -> (w44:cluster{i32, i32})  [unwired: 1 in]
          n298 = Number To Fractional String(number=w233) -> (F-format string=w240:string)  [unwired: 3 in]
          n299 = Increment(x=w98) -> (x+1=w97:i32)
          n300 = call <vilib>:"Excel Easy Text.vi"("report in"=w200, "border? (F)"=FALSE, "font"=w155, "text"=w240, "start (-1, -1)"=w44, "error in (no error)"=w199) -> ("report out"=w198:refnum<class "NI_report.lvclass">, "error out"=w197:errorcluster)  [unwired: 5 in, 3 out]
          n301 = Bundle(w84, w97) -> (w43:cluster{i32, i32})  [unwired: 1 in]
          n302 = Number To Fractional String(number=w231) -> (F-format string=w238:string)  [unwired: 3 in]
          n303 = Increment(x=w97) -> (x+1=w96:i32)
          n304 = call <vilib>:"Excel Easy Text.vi"("report in"=w198, "border? (F)"=FALSE, "font"=w155, "text"=w238, "start (-1, -1)"=w43, "error in (no error)"=w197) -> ("report out"=w196:refnum<class "NI_report.lvclass">, "error out"=w195:errorcluster)  [unwired: 5 in, 3 out]
          n305 = Bundle(w84, w96) -> (w42:cluster{i32, i32})  [unwired: 1 in]
          n306 = Number To Fractional String(number=w154) -> (F-format string=w215:string)  [unwired: 3 in]
          n307 = Increment(x=w96) -> (x+1=w95:i32)
          n308 = call <vilib>:"Excel Easy Text.vi"("report in"=w196, "border? (F)"=FALSE, "font"=w155, "text"=w215, "start (-1, -1)"=w42, "error in (no error)"=w195) -> ("report out"=w194:refnum<class "NI_report.lvclass">, "error out"=w193:errorcluster)  [unwired: 5 in, 3 out]
          n309 = Bundle(w84, w95) -> (w41:cluster{i32, i32})  [unwired: 1 in]
          n310 = Number To Fractional String(number=w153) -> (F-format string=w214:string)  [unwired: 3 in]
          n311 = Increment(x=w95) -> (x+1=w94:i32)
          n312 = call <vilib>:"Excel Easy Text.vi"("report in"=w194, "border? (F)"=FALSE, "font"=w155, "text"=w214, "start (-1, -1)"=w41, "error in (no error)"=w193) -> ("report out"=w192:refnum<class "NI_report.lvclass">, "error out"=w191:errorcluster)  [unwired: 5 in, 3 out]
          n313 = Bundle(w84, w94) -> (w40:cluster{i32, i32})  [unwired: 1 in]
          n314 = Number To Fractional String(number=w152) -> (F-format string=w213:string)  [unwired: 3 in]
          n315 = Increment(x=w94) -> (x+1=w93:i32)
          n316 = call <vilib>:"Excel Easy Text.vi"("report in"=w192, "border? (F)"=FALSE, "font"=w155, "text"=w213, "start (-1, -1)"=w40, "error in (no error)"=w191) -> ("report out"=w190:refnum<class "NI_report.lvclass">, "error out"=w189:errorcluster)  [unwired: 5 in, 3 out]
          n317 = Bundle(w84, w93) -> (w39:cluster{i32, i32})  [unwired: 1 in]
          n318 = Number To Fractional String(number=w151) -> (F-format string=w212:string)  [unwired: 3 in]
          n319 = Increment(x=w93) -> (x+1=w92:i32)
          n320 = call <vilib>:"Excel Easy Text.vi"("report in"=w190, "border? (F)"=FALSE, "font"=w155, "text"=w212, "start (-1, -1)"=w39, "error in (no error)"=w189) -> ("report out"=w188:refnum<class "NI_report.lvclass">, "error out"=w187:errorcluster)  [unwired: 5 in, 3 out]
          n321 = Bundle(w84, w92) -> (w38:cluster{i32, i32})  [unwired: 1 in]
          n322 = Number To Fractional String(number=w150) -> (F-format string=w211:string)  [unwired: 3 in]
          n323 = Increment(x=w92) -> (x+1=w91:i32)
          n324 = call <vilib>:"Excel Easy Text.vi"("report in"=w188, "border? (F)"=FALSE, "font"=w155, "text"=w211, "start (-1, -1)"=w38, "error in (no error)"=w187) -> ("report out"=w186:refnum<class "NI_report.lvclass">, "error out"=w185:errorcluster)  [unwired: 5 in, 3 out]
          n325 = Bundle(w84, w91) -> (w37:cluster{i32, i32})  [unwired: 1 in]
          n326 = Number To Fractional String(number=w149) -> (F-format string=w210:string)  [unwired: 3 in]
          n327 = Increment(x=w91) -> (x+1=w90:i32)
          n328 = call <vilib>:"Excel Easy Text.vi"("report in"=w186, "border? (F)"=FALSE, "font"=w155, "text"=w210, "start (-1, -1)"=w37, "error in (no error)"=w185) -> ("report out"=w184:refnum<class "NI_report.lvclass">, "error out"=w183:errorcluster)  [unwired: 5 in, 3 out]
          n329 = Bundle(w84, w90) -> (w36:cluster{i32, i32})  [unwired: 1 in]
          n330 = Number To Fractional String(number=w148) -> (F-format string=w209:string)  [unwired: 3 in]
          n331 = Increment(x=w90) -> (x+1=w89:i32)
          n332 = call <vilib>:"Excel Easy Text.vi"("report in"=w184, "border? (F)"=FALSE, "font"=w155, "text"=w209, "start (-1, -1)"=w36, "error in (no error)"=w183) -> ("report out"=w182:refnum<class "NI_report.lvclass">, "error out"=w181:errorcluster)  [unwired: 5 in, 3 out]
          n333 = Bundle(w84, w89) -> (w35:cluster{i32, i32})  [unwired: 1 in]
          n334 = Number To Fractional String(number=w147) -> (F-format string=w208:string)  [unwired: 3 in]
          n335 = Increment(x=w89) -> (x+1=w88:i32)
          n336 = call <vilib>:"Excel Easy Text.vi"("report in"=w182, "border? (F)"=FALSE, "font"=w155, "text"=w208, "start (-1, -1)"=w35, "error in (no error)"=w181) -> ("report out"=w180:refnum<class "NI_report.lvclass">, "error out"=w179:errorcluster)  [unwired: 5 in, 3 out]
          n337 = Bundle(w84, w88) -> (w34:cluster{i32, i32})  [unwired: 1 in]
          n338 = Number To Fractional String(number=w146) -> (F-format string=w207:string)  [unwired: 3 in]
          n339 = Increment(x=w88) -> (x+1=w87:i32)
          n340 = call <vilib>:"Excel Easy Text.vi"("report in"=w180, "border? (F)"=FALSE, "font"=w155, "text"=w207, "start (-1, -1)"=w34, "error in (no error)"=w179) -> ("report out"=w178:refnum<class "NI_report.lvclass">, "error out"=w177:errorcluster)  [unwired: 5 in, 3 out]
          n341 = Bundle(w84, w87) -> (w33:cluster{i32, i32})  [unwired: 1 in]
          n342 = Number To Fractional String(number=w145) -> (F-format string=w206:string)  [unwired: 3 in]
          n343 = Increment(x=w87) -> (x+1=w86:i32)
          n344 = call <vilib>:"Excel Easy Text.vi"("report in"=w178, "border? (F)"=FALSE, "font"=w155, "text"=w206, "start (-1, -1)"=w33, "error in (no error)"=w177) -> ("report out"=w176:refnum<class "NI_report.lvclass">, "error out"=w175:errorcluster)  [unwired: 5 in, 3 out]
          n345 = Bundle(w84, w86) -> (w32:cluster{i32, i32})  [unwired: 1 in]
          n346 = Number To Fractional String(number=w144) -> (F-format string=w205:string)  [unwired: 3 in]
          n347 = Increment(x=w86) -> (x+1=w85:i32)
          n348 = call <vilib>:"Excel Easy Text.vi"("report in"=w176, "border? (F)"=FALSE, "font"=w155, "text"=w205, "start (-1, -1)"=w32, "error in (no error)"=w175) -> ("report out"=w174:refnum<class "NI_report.lvclass">, "error out"=w173:errorcluster)  [unwired: 5 in, 3 out]
          n349 = Bundle(w84, w85) -> (w31:cluster{i32, i32})  [unwired: 1 in]
          n350 = Number To Fractional String(number=w143) -> (F-format string=w204:string)  [unwired: 3 in]
          n351 = Increment(x=w85) -> (x+1=w82:i32)
          n352 = call <vilib>:"Excel Easy Text.vi"("report in"=w174, "border? (F)"=FALSE, "font"=w155, "text"=w204, "start (-1, -1)"=w31, "error in (no error)"=w173) -> ("report out"=w172:refnum<class "NI_report.lvclass">, "error out"=w171:errorcluster)  [unwired: 5 in, 3 out]
          n353 = Bundle(w84, w82) -> (w30:cluster{i32, i32})  [unwired: 1 in]
          n354 = Number To Fractional String(number=w142) -> (F-format string=w203:string)  [unwired: 3 in]
          n355 = Increment(x=w82) -> (x+1=w83:i32)
          n356 = call <vilib>:"Excel Easy Text.vi"("report in"=w172, "border? (F)"=FALSE, "font"=w155, "text"=w203, "start (-1, -1)"=w30, "error in (no error)"=w171) -> ("report out"=w170:refnum<class "NI_report.lvclass">, "error out"=w169:errorcluster)  [unwired: 5 in, 3 out]
          n357 = Bundle(w84, w83) -> (w29:cluster{i32, i32})  [unwired: 1 in]
          n358 = Number To Fractional String(number=w141) -> (F-format string=w202:string)  [unwired: 3 in]
          n359 = call <vilib>:"Excel Easy Text.vi"("report in"=w170, "border? (F)"=FALSE, "font"=w155, "text"=w202, "start (-1, -1)"=w29, "error in (no error)"=w169) -> ("report out"=w140:refnum<class "NI_report.lvclass">, "error out"=w139:errorcluster)  [unwired: 5 in, 3 out]
          n360 = call <vilib>:"Excel Get ActiveX References.vi"("report in"=w140, "error in (no error)"=w139) -> ("Excel._Workbook"=w23:refnum<k7>, "error out"=w22:errorcluster)  [unwired: 12 out]
          n361 = invoke class="_Workbook" method="SaveAs"(reference=w23, error in=w22, "Filename"=w21) -> (error out=→"error out 2":errorcluster)  [unwired: 13 in, 15 out]
        }
      }
    }
  }
